vi "WPI_CAN_PDPDecode4Currents.vi"(10 "5-Byte Array":u8[](array[numeric])) -> (2 "4-Current Array":dbl[](array[numeric]))   [LabVIEW 2017]
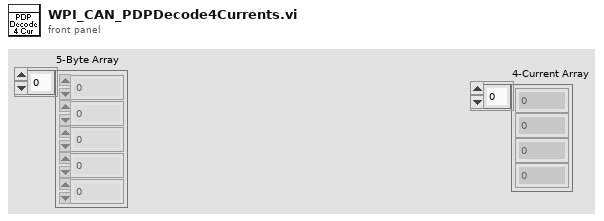
[diagram p1: front panel]
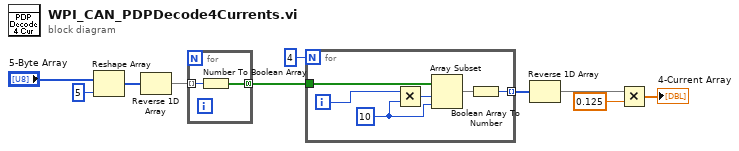
[diagram p0: block diagram]
diagram:
  n1 = Reshape Array("5-Byte Array", 5 ("dimension size")) -> (w2:u8[])
  n2 = Reverse 1D Array(array=w2) -> (reversed array=w10:u8[])
  n3 = for {
    tunnel: w10 -> [w12] mode=indexing
    tunnel: [w11] -> w8 mode=concatenating
    n4 = Number To Boolean Array(number=w12) -> (Boolean array=w11:bool[])
  }
  n5 = for {
    N: 4 -> [_]
    tunnel: w8 -> [w18]
    tunnel: [w13] -> w7 mode=indexing
    i -> [w16]
    w15 = 10 ("length")
    n6 = Multiply(x=w16, y=w15) -> (x*y=w17:i32)
    n7 = Array Subset(array=w18, index=w17, length=w15) -> (w14:bool[])
    n8 = Boolean Array To Number(Boolean array=w14) -> (number=w13:u32)
  }
  n9 = Reverse 1D Array(array=w7) -> (reversed array=w5:u32[])
  n10 = Multiply(x=w5, y=0.125) -> (x*y=→"4-Current Array":dbl[])
